vi "Append to Service Map.vi"(8 "error in":errorcluster, 10 "Map Entry":T1={"CobID"=0, "Data offset"=4, "Data size"=4, "Destination"=refnum}, 11 "CAN Task in":refnum<class "CAN Task.lvclass">) -> (0 "error out":errorcluster, 3 "CAN Task out":refnum<class "CAN Task.lvclass">)   [LabVIEW 2024, in "canopen.lvlib" / "CAN Task.lvlib" / "CAN Task.lvclass"]
uses:
  CAN Task.lvclass
  CAN Task.lvclass/CAN Task.ctl
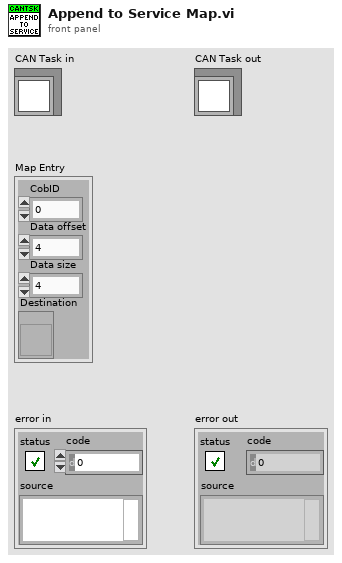
[diagram p1: front panel]
types:
  T1 = cluster{"CobID":u32, "Data offset":u8, "Data size":u8, "Destination":refnum<vi>}
  T2 = cluster{"CobID":u32, "Data offset":u8, "Data size":u8, "Destination":refnum<vi>}[]
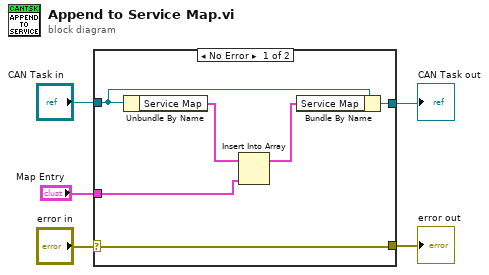
[diagram p0: block diagram]
diagram:
  n1 = case shown="No Error" "error in" {
    selector: "error in" -> [w6 w13]
    tunnel: [w6 w13] -> w5
    tunnel: "CAN Task in" -> [w11 w12]
    tunnel: "Map Entry" -> [w9 _]
    tunnel: [w7 w12] -> w1
    frame No Error {
      n2 = Unbundle By Name(w11) -> ("Service Map"=w10:T2)
      n3 = Insert Into Array(array=w10, new element=w9) -> (w8:T2)  [unwired: 1 in]
      n4 = Bundle By Name(cluster=w11, "Service Map"=w8) -> (w7:refnum<class "CAN Task.lvclass">)
    }
    frame Error {
    }
  }
  "error out" <- w5
  "CAN Task out" <- w1
